vi "Read Allow Undefined Strings.vi"(8 "error in (no error)":errorcluster, 11 "ComboBox.lvclass in":refnum<class "ComboBox.lvclass">) -> (0 "error out":errorcluster, 2 "AllowUndefStrs":bool, 3 "ComboBox.lvclass out":refnum<class "ComboBox.lvclass">)   [LabVIEW 2015, in "ComboBox.lvclass"]
uses:
  ComboBox.lvclass
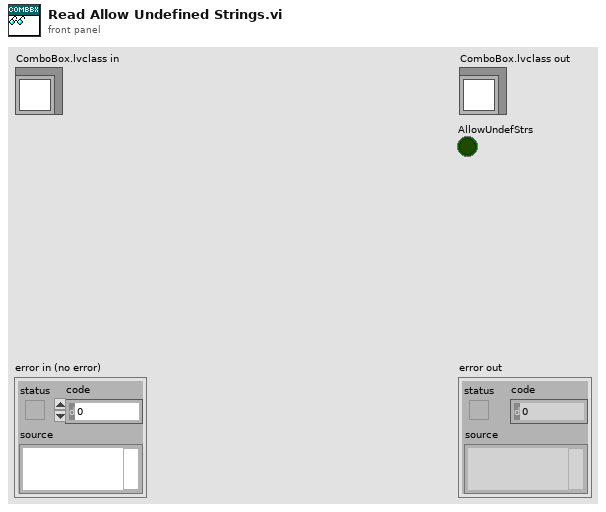
[diagram p1: front panel]
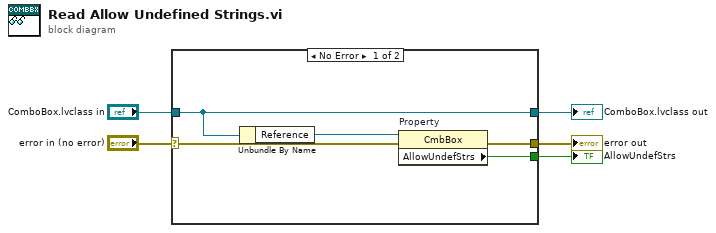
[diagram p0: block diagram]
diagram:
  n1 = case shown="No Error" "error in (no error)" {
    selector: "error in (no error)" -> [w6 w12]
    tunnel: [w9 w12] -> w4
    tunnel: [w8 w11] -> w2
    tunnel: "ComboBox.lvclass in" -> [w8 w11]
    tunnel: [w10 _] -> w1
    frame No Error {
      n2 = Unbundle By Name(w8) -> ("Reference"=w7:refnum<vi>)
      n3 = property on="Property" class="CmbBox"(reference=w7, error in=w6) -> (error out=w9:errorcluster, "AllowUndefStrs"=w10:bool)  [unwired: 1 out]
    }
    frame Error {
    }
  }
  "error out" <- w4
  "ComboBox.lvclass out" <- w2
  "AllowUndefStrs" <- w1
